vi "Load Config_Main.vi"(8 "error in (no error)":errorcluster, 11 "Refnum in":T1) -> (0 "error out":errorcluster, 2 "Main":T2, 3 "Refnum out":T1)   [LabVIEW 2019, in "AutoMenuCreator.lvlib"]
uses:
  AutoMenuCreator.lvlib
  Ctl/Ctl_Config_Main.ctl
  <vilib>/Utility/config.llb/Config Data RefNum.ctl
  <vilib>/Utility/config.llb/NI_LVConfig.lvlib
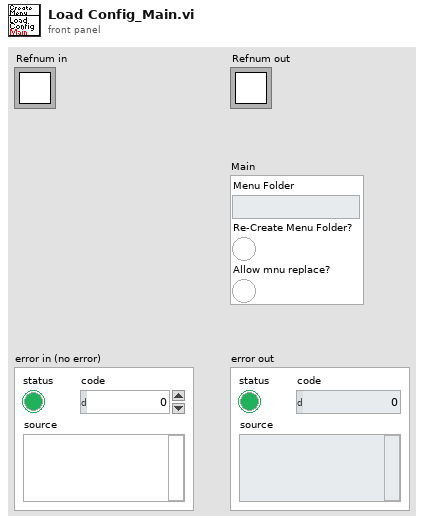
[diagram p1: front panel]
types:
  T1 = typedef "NI_LVConfig.lvlib/Config Data RefNum.ctl" = refnum<k1>
  T2 = typedef "AutoMenuCreator.lvlib/Ctl_Config_Main.ctl" = cluster{"Menu Folder":string, "Re-Create Menu Folder?":bool, "Allow mnu replace?":bool}
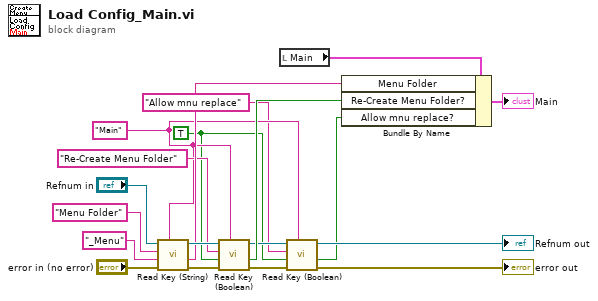
[diagram p0: block diagram]
diagram:
  w4 = TRUE
  w6 = "Main" ("section")
  n1 = call <vilib>:"Read Key (String).vi"("section"=w6, "error in (no error)"="error in (no error)", "default value"="_Menu", "key"="Menu Folder", "refnum"="Refnum in") -> ("error out"=w18:errorcluster, "value"=w15:string, "refnum out"=w19:T1)  [unwired: 3 in, 1 out]
  n2 = call <vilib>:"Read Key (Boolean).vi"("section"=w6, "error in (no error)"=w18, "default value"=w4, "key"="Re-Create Menu Folder", "refnum"=w19) -> ("error out"=w5:errorcluster, "value"=w14:bool, "refnum out"=w8:T1)  [unwired: 3 in, 1 out]
  n3 = local read "Main"() -> (w9:T2)
  n4 = call <vilib>:"Read Key (Boolean).vi"("section"=w6, "error in (no error)"=w5, "default value"=w4, "key"="Allow mnu replace", "refnum"=w8) -> ("error out"=→"error out":errorcluster, "value"=w3:bool, "refnum out"=→"Refnum out":T1)  [unwired: 3 in, 1 out]
  n5 = Bundle By Name(cluster=w9, "Menu Folder"=w15, "Re-Create Menu Folder?"=w14, "Allow mnu replace?"=w3) -> (→"Main":T2)
